vi "toVector.vi"(10 "Y Component":dbl, 11 "X Component":dbl) -> (3 "Vector <x,y>":dbl[](array[numeric]))   [LabVIEW 2015]
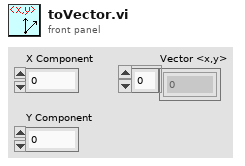
[diagram p1: front panel]
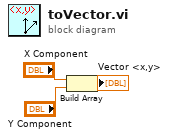
[diagram p0: block diagram]
diagram:
  n1 = Build Array("X Component", "Y Component") -> (→"Vector <x,y>":dbl[])
